vi "Radians_To_Degrees.vi"(10 "Radians":dbl) -> (2 "Degrees":dbl)   [LabVIEW 2011]
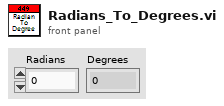
[diagram p1: front panel]
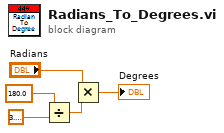
[diagram p0: block diagram]
diagram:
  n1 = Divide(x=180.0 ("y"), y=3.141592653589793) -> (x/y=w5:dbl)
  n2 = Multiply(x="Radians", y=w5) -> (x*y=→"Degrees":dbl)
